vi "CountAtomsFast.vi"(8 "Experimental Variables":T1={"Pixel Size before binning (µm)"=6.0, "Imaging Wavelength (m)"=4.61e-07, "Isotope"=84, "1P1 Linewidth (MHz)"=30.5, "Imaging Detuning (MHz)"=0.0, "Software Bin Size"=1, "Exp. Trigger ON time (ms)"=0.0, "Path to spinapi.dll"=path "C:/SpinCore/SpinAPI/lib32/spinapi.dll", "PB clock_freq (MHz)"=100.0} {"Software Bin Size" items=["1"=1, "2"=2, "3"=3, "4"=4, "5"=5, "6"=6, "7"=7, "8"=8]; "Isotope" min=84 max=88; "Imaging Wavelength (m)" format="%#_6p"}, 9 "Background Image":dbl[][](graph), 10 "Atom Image":dbl[][](graph), 11 "Cursor List":T2) -> (0 "Data Cuts":dbl[][](graph), 1 "OD":dbl[][](graph), 2 "Number":dbl)   [LabVIEW 2016]
uses:
  <vilib>/Utility/miscctls.llb/LVCursorListTypeDef.ctl
  Controls/ExperimentParameters/experimentalvariables.ctl
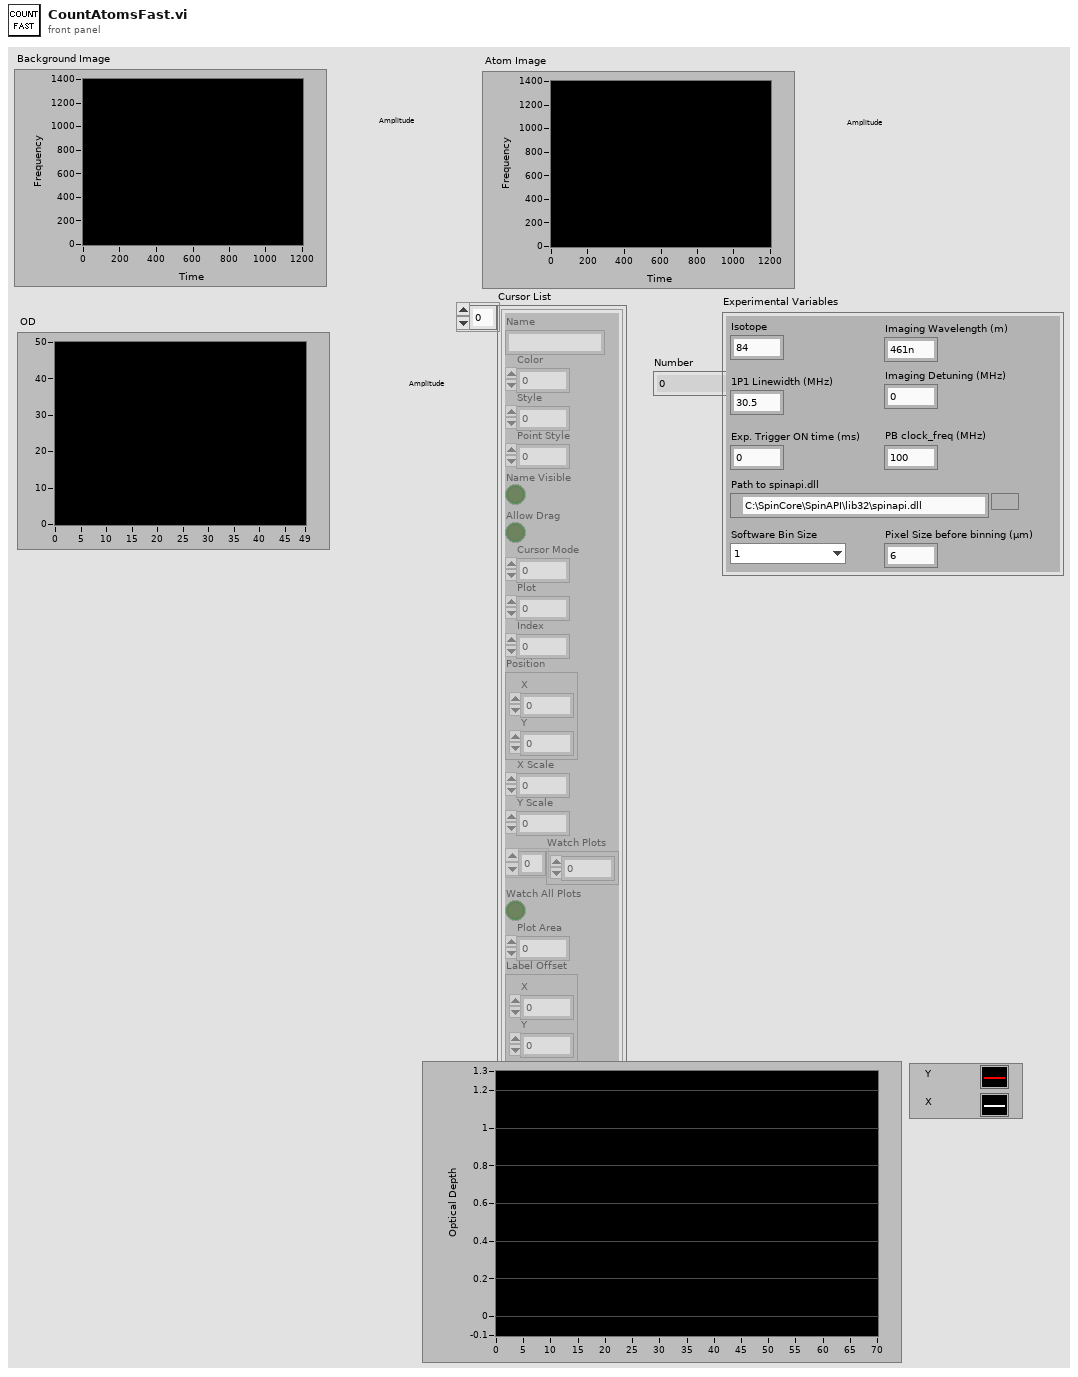
[diagram p1: front panel]
types:
  T1 = typedef "experimentalvariables.ctl" = cluster{"Pixel Size before binning (µm)":dbl, "Imaging Wavelength (m)":dbl, "Isotope":i32, "1P1 Linewidth (MHz)":dbl, "Imaging Detuning (MHz)":dbl, "Software Bin Size":u16, "Exp. Trigger ON time (ms)":dbl, "Path to spinapi.dll":path, "PB clock_freq (MHz)":dbl}
  T2 = typedef "LVCursorListTypeDef.ctl" = cluster{"Name":string, "Color":u32, "Style":u8, "Point Style":u8, "Name Visible":bool, "Allow Drag":bool, "Cursor Mode":u32, "Plot":i32, "Index":i32, "Position":cluster{"X":dbl, "Y":dbl}, "X Scale":u32, "Y Scale":u32, "Watch Plots":i32[], "Watch All Plots":bool, "Plot Area":i32, "Label Offset":cluster{"X":dbl, "Y":dbl}}[]
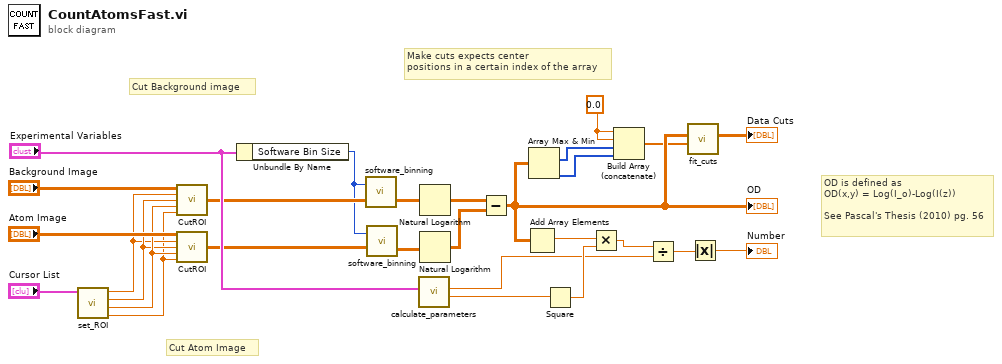
[diagram p0: block diagram]
diagram:
  w8 = 0.0 ("element")
  # "Make cuts expects center \npositions in a certain index of the array"
  # "OD is defined as \nOD(x,y) = Log(I_o)-Log(I(z))\n\nSee Pascal's Thesis (2010) pg. 56"
  # "Cut Atom Image"
  # "Cut Background image"
  n1 = call "set_ROI.vi"("Cursor List"="Cursor List") -> ("Row End"=w15:dbl, "RowStart"=w23:dbl, "ColEnd"=w22:dbl, "ColStart"=w21:dbl)  [unwired: 7 in]
  n2 = call "CutROI.vi"("Full Image In"="Background Image", "Col Start"=w21, "Col End"=w22, "Row Start"=w23, "Row End"=w15) -> ("Cut Image Out"=w13:dbl[][])  [unwired: 10 in]
  n3 = call "CutROI.vi"("Full Image In"="Atom Image", "Col Start"=w21, "Col End"=w22, "Row Start"=w23, "Row End"=w15) -> ("Cut Image Out"=w11:dbl[][])  [unwired: 10 in]
  n4 = Unbundle By Name("Experimental Variables") -> ("Software Bin Size"=w9:u16)
  n5 = call "software_binning.vi"("Input Array"=w13, "bin size"=w9) -> ("Binned Array"=w12:dbl[][])  [unwired: 1 in]
  n6 = call "software_binning.vi"("Input Array"=w11, "bin size"=w9) -> ("Binned Array"=w10:dbl[][])  [unwired: 1 in]
  n7 = call "calculate_parameters.vi"("Experimental Variables"="Experimental Variables") -> ("Effective Pixel Size (µm)"=w17:dbl, "Cross Section (m^2)"=w16:dbl)  [unwired: 8 in, 1 out]
  n8 = Natural Logarithm(1:w12) -> (0:w25:dbl[][])
  n9 = Natural Logarithm(1:w10) -> (0:w24:dbl[][])
  n10 = Subtract(x=w25, y=w24) -> (x-y=w5:dbl[][])
  "OD" <- w5
  n11 = Add Array Elements(numeric array=w5) -> (sum=w20:dbl)
  n12 = Array Max & Min(array=w5) -> (max index (indices)=w7:i32[], min index (indices)=w6:i32[])  [unwired: 2 out]
  n13 = Square(x=w17) -> (x^2=w18:dbl)
  n14 = Multiply(x=w20, y=w18) -> (x*y=w19:dbl)
  n15 = Build Array (concatenate)(w8, w8, w7, w6) -> (w4:dbl[])
  n16 = Divide(x=w19, y=w16) -> (x/y=w2:dbl)
  n17 = call "fit_cuts.vi"("Array"=w4, "Intensity Graph"=w5) -> ("Waveform Graph"=→"Data Cuts":dbl[][])  [unwired: 9 in]
  n18 = Absolute Value(x=w2) -> (abs(x)=→"Number":dbl)
